vi "Shutdown Master.vi"(8 "error in (no error)":errorcluster, 11 "TCP master in":refnum<class "TCP Master.lvclass">) -> (0 "error out":errorcluster, 3 "TCP master out":refnum<class "TCP Master.lvclass">)   [LabVIEW 2018, in "SubVIs.lvlib" / "TCP Master.lvclass"]
doc: "Closes the TCP connection stored in the class."
uses:
  TCP Master.lvclass
  TCP Master.lvclass/TCP Master.ctl
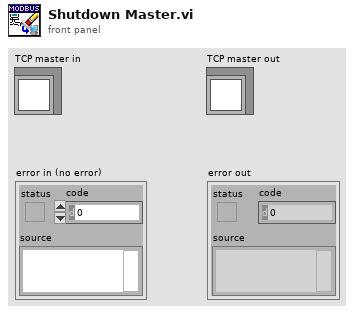
[diagram p1: front panel]
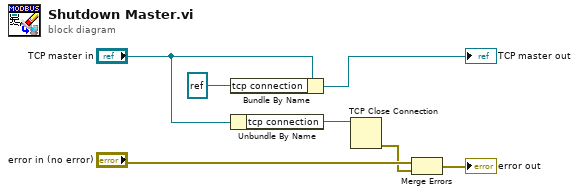
[diagram p0: block diagram]
diagram:
  n1 = Bundle By Name(cluster="TCP master in", "tcp connection"=refnum<k5> refnum) -> (→"TCP master out":refnum<class "TCP Master.lvclass">)
  n2 = Unbundle By Name("TCP master in") -> ("tcp connection"=w5:refnum<k5>)
  n3 = TCP Close Connection(connection ID=w5) -> (error out=w2:errorcluster)  [unwired: 2 in, 1 out]
  n4 = Merge Errors("error in (no error)", w2) -> (→"error out":errorcluster)
